vi "Update.vi"(8 "error in (no error)":errorcluster caption="entrée d'erreur (pas d'erreur)", 11 "Timed Loop Controller en entrée":refnum<class "Timed Loop Controller.lvclass">) -> (0 "error out":errorcluster caption="sortie d'erreur", 3 "Timed Loop Controller en sortie":refnum<class "Timed Loop Controller.lvclass">)   [LabVIEW 2015, in "Timed Loop Controller.lvlib" / "Timed Loop Controller.lvclass"]
uses:
  Timed Loop Controller.lvclass
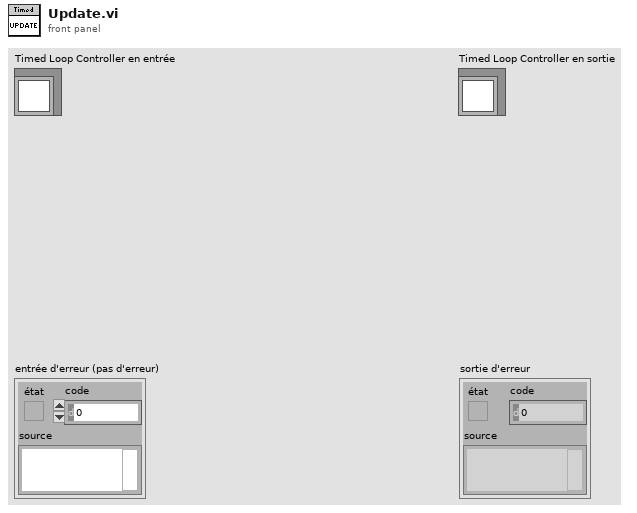
[diagram p1: front panel]
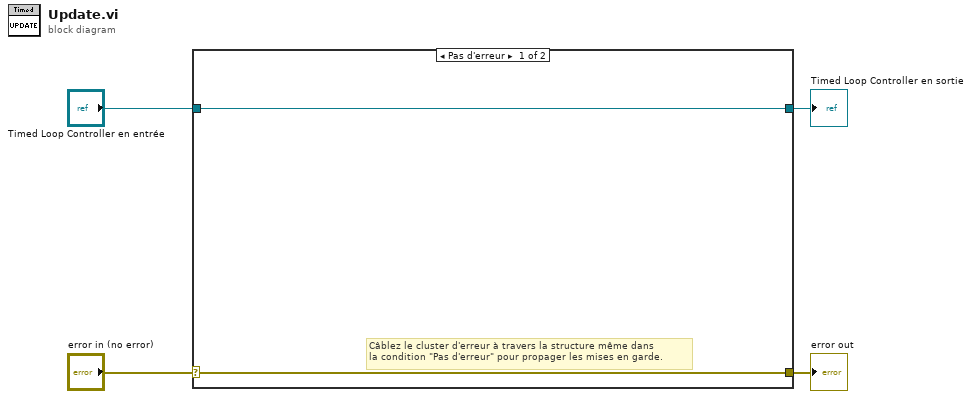
[diagram p0: block diagram]
diagram:
  n1 = case shown="Pas d'erreur" "error in (no error)" {
    selector: "error in (no error)" -> [w5 w8]
    tunnel: [w5 w8] -> w3
    tunnel: [w6 w7] -> w1
    tunnel: "Timed Loop Controller en entrée" -> [w6 w7]
    frame No Error {
      # "Câblez le cluster d'erreur à travers la structure même dans\nla condition \"Pas d'erreur\" pour propager les mises en garde."
    }
    frame Error {
    }
  }
  "error out" <- w3
  "Timed Loop Controller en sortie" <- w1
